vi "PDF Protokoll EPA1065_308 T90.vi"(8 "error in (no error)":errorcluster caption="Fehler (Eingang, kein Fehler)") -> (0 "error out":errorcluster caption="Fehler (Ausgang)")   [LabVIEW 2020, in "EPA 1065.lvlib" / "T90 Test 1065-308.lvlib"]
uses:
  T90 Test 1065-308.lvlib
  Ergebnis.ctl
  Modus.ctl
  Aktion FGV T90.ctl
  Seiten/FT-IR/FGV FT-IR Gasliste Aktionen.ctl
  Seiten/FT-IR/FGV FT-IR Aktionen.ctl
  Seiten/System Einstellungen V2/Aktioen FGV System Konstanten.ctl
  Sprachverwaltung/FGV Aktion Tabelle zerlegen.ctl
  Aktion FGV Datenmanagment.ctl
  Seiten/Anlagengrenzwerte/FGV Anlagengrenzwerte Aktionen.ctl
  <vilib>/Utility/miscctls.llb/LVPrintingMarginsTypeDef.ctl
  Allgemein/allgemeine Sub-VIs.lvlib
  Seiten/FT-IR/FT-IR.lvlib
  Seiten/System Einstellungen V2/System Einstellungen V2.lvlib
  Seiten/Anlagengrenzwerte/Anlagengrenzwerte.lvlib
  Sprachverwaltung/Sprachverwaltung.lvlib
panel:
  out "Modus":string caption="Mode:"
  in  "Modus":T1 caption="Modus:" items=["CG zu PNS", "CG zu Entnahmestelle"]
  out "Einheit 2":string caption="Einheit"
  out "Durchfluss FT-IR:":string caption="Flow FTIR:"
  out "Frequenz 2":string
  out "Frequenz 1":string
  out "Versa Serial number:":string caption="Serial number:"
  out "Anlage:":string caption="Measuring Device:"
  out "Methode (Recipe):":string
  out "Date & Time:":string
  out "Accuracy:":string
  out "Gas Bottle Nr.:":string
  out "Ergebnis 4":T2
  out "Ergebnis 3":T2
  out "Ergebnis 2":T2
  out "Ergebnis 1":T2
  out "Averaged T90-T10 2":string caption="Averaged T90-T10"
  out "Averaged T10-T90 2":string caption="Averaged T10-T90"
  out "Ergebnis x5 (T90 T10)":string caption="Mean T10-T90"
  out "Ergebnis x5 (T10 T90)":string caption="Mean T10-T90"
  out "Averaged T90-T10":string
  out "Averaged T10-T90":string
  out "T90 Result":waveform(sgl)(graph) caption="T90"
  out "Tabelle":string[][](table)
  out "Ergebnis:":string caption="Result:"
  out "Konzentration:":string caption="Setpoint:"
  out "Komponente:":string caption="Component:"
  out "Bearbeiter:":string caption="Editor:"
  out "Serial number:":string
  out "Messgerät:":string caption="Analyzer:"
  # "T90 EPA § 1065.308"
  # "Limits"
  # "Result"
  # "s"
  # ">5"
  # "s"
  # ">5"
  # "s"
  # "<10s"
  # "s"
  # "<10s"
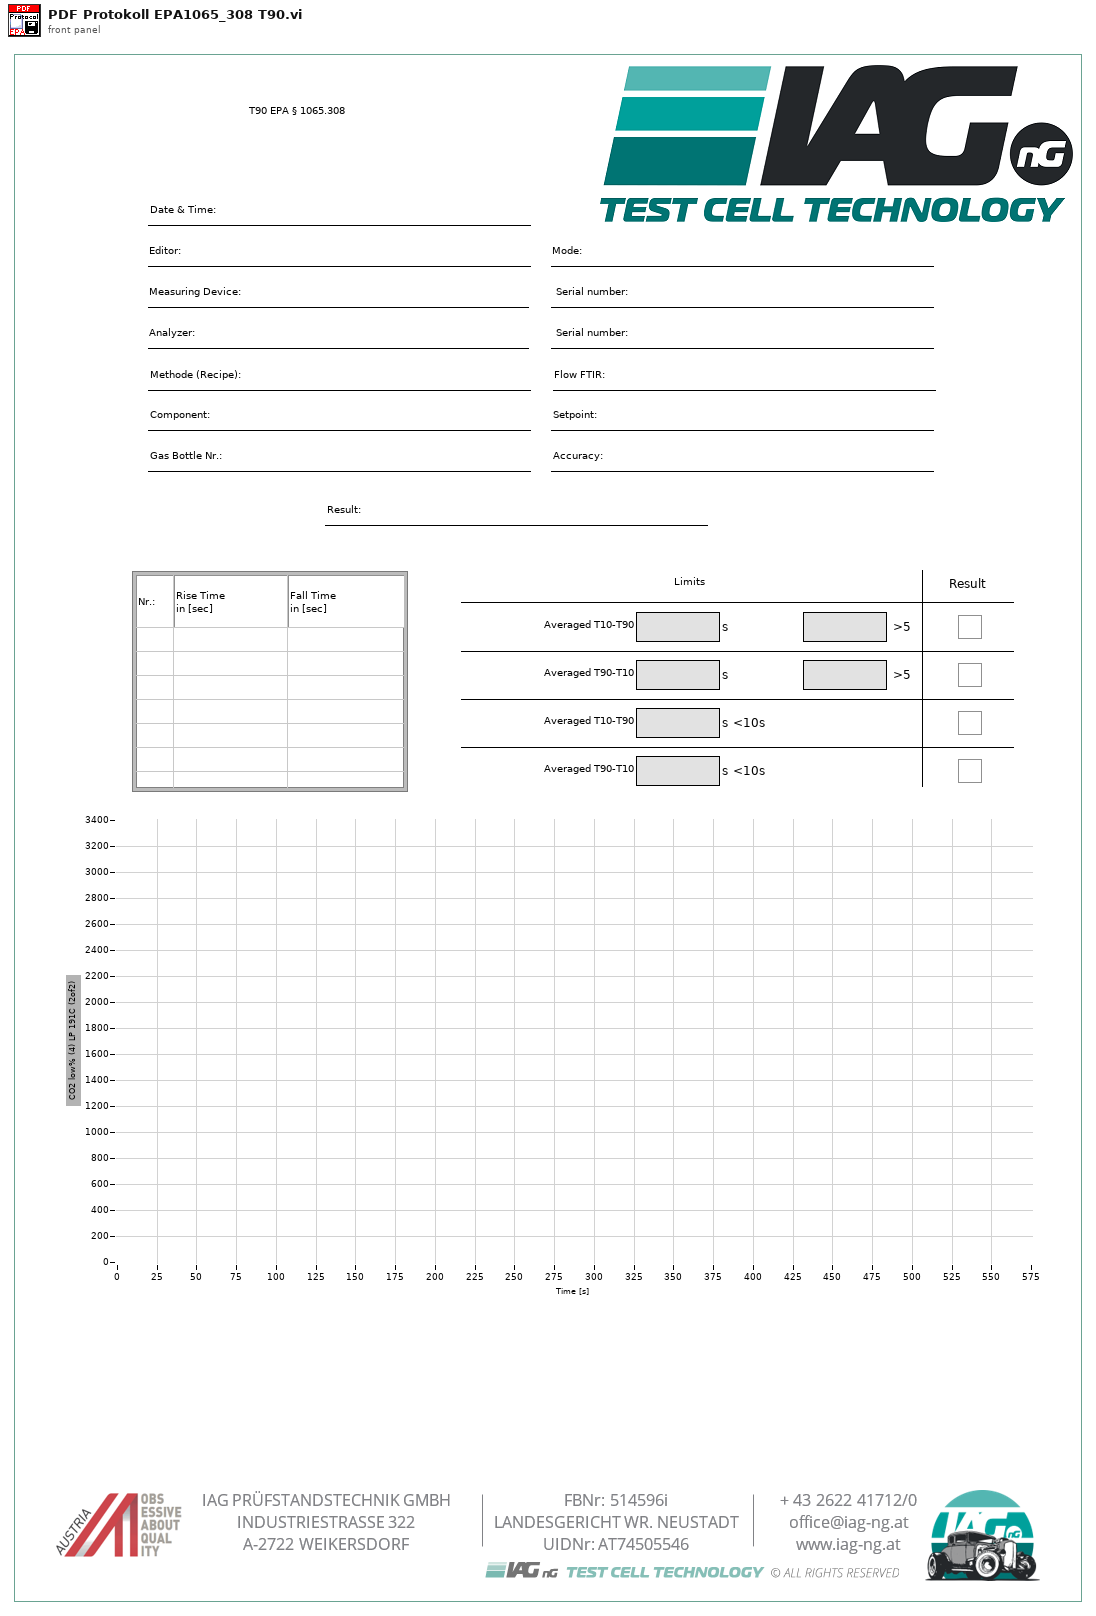
[diagram p1: front panel]
types:
  T1 = typedef "EPA 1065.lvlib/T90 Test 1065-308.lvlib/Modus.ctl" = u16
  T2 = typedef "EPA 1065.lvlib/T90 Test 1065-308.lvlib/Ergebnis.ctl" = bool
  T3 = typedef "Sprachverwaltung.lvlib/FGV Aktion Tabelle zerlegen.ctl" = enum16{"laden", "vereinzeln", "speichern"}
  T4 = typedef "System Einstellungen V2.lvlib/Aktioen FGV System Konstanten.ctl" = enum16{"lesen", "laden", "speichern", "Sprache"}
  T5 = typedef "FT-IR.lvlib/FGV FT-IR Aktionen.ctl" = enum16{"lesen", "NOG setzen", "NOS setzen", "Initialisieren", "speichern", "ALLES setzen", "FT-IR Spektrum loggen", "Komm Stoppen", "Spektrum LogKonfig"}
  T6 = typedef "FT-IR.lvlib/FGV FT-IR Gasliste Aktionen.ctl" = enum16{"lesen", "Gasliste FT-IR", "Gasliste ausgelesen", "laden", "speichern", "löschen"}
  T7 = typedef "EPA 1065.lvlib/T90 Test 1065-308.lvlib/Aktion FGV T90.ctl" = enum16{"lesen", "Konfig Daten", "speichern", "laden", "T90 aktiv", "T90 inaktiv", "Ext. Ventil aktivieren", "Ext. Ventil deaktivieren", "N2 spülen aktiv", "N2 spülen inaktiv", "Ergebnis Textfile"}
  T8 = typedef "EPA 1065.lvlib/T90 Test 1065-308.lvlib/Aktion FGV Datenmanagment.ctl" = enum16{"init", "lesen", "Istwerte schreiben", "höchsten Peak setzen", "Auswerten", "Grenzen setzen", "Sollwert ändern", "Rise T10", "Rise T90", "Fall T90", "Fall T10", "Bit löschen", "Umschaltzeitpunkt"}
  T9 = typedef "Anlagengrenzwerte.lvlib/FGV Anlagengrenzwerte Aktionen.ctl" = enum16{"Lesen", "Grenzwerte schreiben"}
  T10 = enum32{"Portrait", "Landscape", "Rotated Portrait", "Rotated Landscape"}
  T11 = typedef "LVPrintingMarginsTypeDef.ctl" = cluster{"Top":sgl, "Left":sgl, "Bottom":sgl, "Right":sgl, "Measurement System":enum8{"Inches", "cm"}}
  T12 = typedef "EPA 1065.lvlib/T90 Test 1065-308.lvlib/T90 Konfig Daten.ctl" = cluster{"Bearbeiter:":string, "Komponente:":u16, "Gasflaschen Nr.:":string, "Accuracy":dbl, "Sollwert":dbl, "Modus":T1, "Abschaltzeit:":dbl, "Abweichung:":dbl, "Pfad:":path, "Textname:":string, "CG Aufschaltzeit:":dbl, "Einheit":string, "N2 Aufschaltzeit:":dbl, "Analysator":T13, "Gasflasche":T14, "Konfig Gasflasche":T15, "Frequency:":T16}
  T13 = typedef "System Einstellungen V2.lvlib/Analysatoren.ctl" = string
  T14 = typedef "System Einstellungen V2.lvlib/Gasflasche Auswahl.ctl" = u16
  T15 = typedef "System Einstellungen V2.lvlib/Konfig Gasflasche.ctl" = bool
  T16 = typedef "EPA 1065.lvlib/T90 Test 1065-308.lvlib/Frequenz.ctl" = u16
  T17 = cluster{"Modell":string, "ProjektNummer":string, "Software Version":string, "Seriennummer":string}
  T18 = typedef "String - Ausgabefeld.ctl" = string
  T19 = typedef "EPA 1065.lvlib/T90 Test 1065-308.lvlib/Datencluster.ctl" = cluster{"Höchster Peak":T20, "T10 Grenzwert":T20, "T90 Grenzwert":T20, "Rise Times":dbl[], "Fall Times":dbl[], "RiseTime gemittelt":T20, "FallTime gemittelt":T20, "Zeitstempel":timestamp[], "Rise T10":bool, "Rise T90":bool, "Fall T10":bool, "Fall T90":bool, "RiseTime >5":bool, "Falltime >5":bool, "RiseTime <10":bool, "Falltime <10":bool, "T0-T90":dbl[], "T100-T10":dbl[]}
  T20 = typedef "Zahlen-Eingabefeld.ctl" = sgl
  T21 = typedef "Anlagengrenzwerte.lvlib/Anlagen-Grenzwerte Anzeige.ctl" = cluster{"Eingangsdruck FT-IR:":T22, "Durchfluss FT-IR:":T22, "Durchfluss CalGas:":T22, "Druck Ausgang:":T22, "Druck Kalter Block:":T22, "Heizleitungen intern:":T22, "Heizleitung zu FT-IR:":T22, "Heizung Filterblock:":T22, "Heizung Pumpe:":T22, "Heizleitung Extern SP1:":T22, "Heizleitung Extern SP2:":T22, "FT-IR Heizung Messzelle:":T22, "Schaltschranktemperatur:":T22, "Gaskühler:":T22}
  T22 = typedef "Anlagengrenzwerte.lvlib/Anlagen-Parameter Anzeige.ctl" = cluster{"Sollwert":sgl, "Warn-Min":sgl, "Warn-Max":sgl, "Abschalt-Min":sgl, "Abschalt-Max":sgl, "Regler":u16}
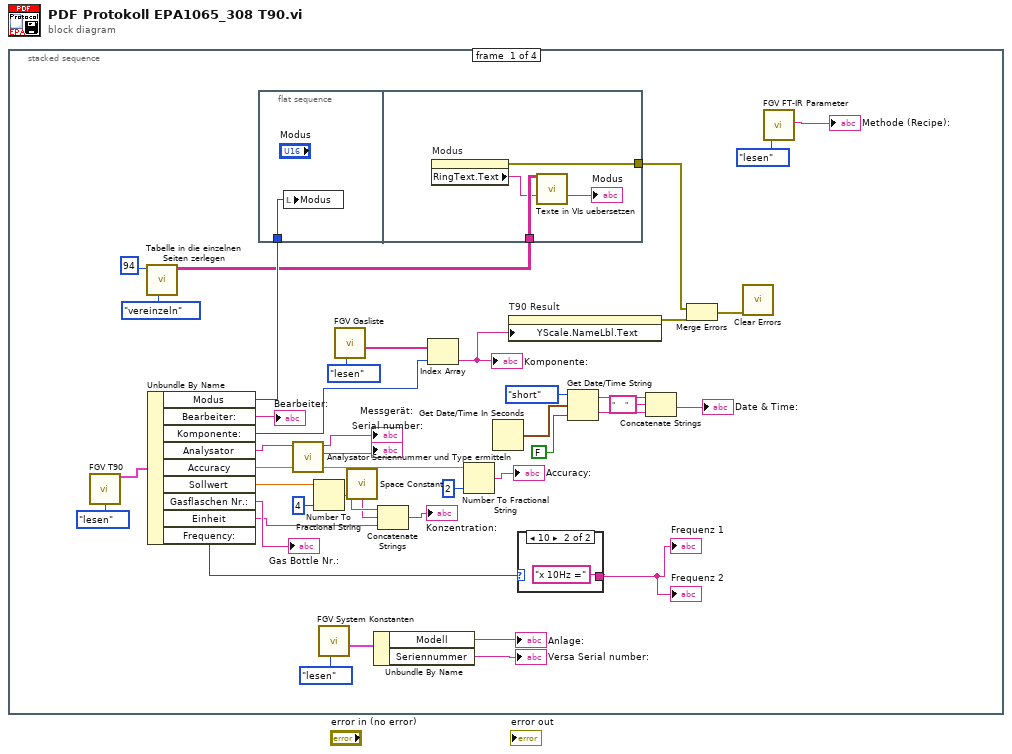
[diagram p0: block diagram]
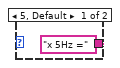
[diagram p2: hidden frame]
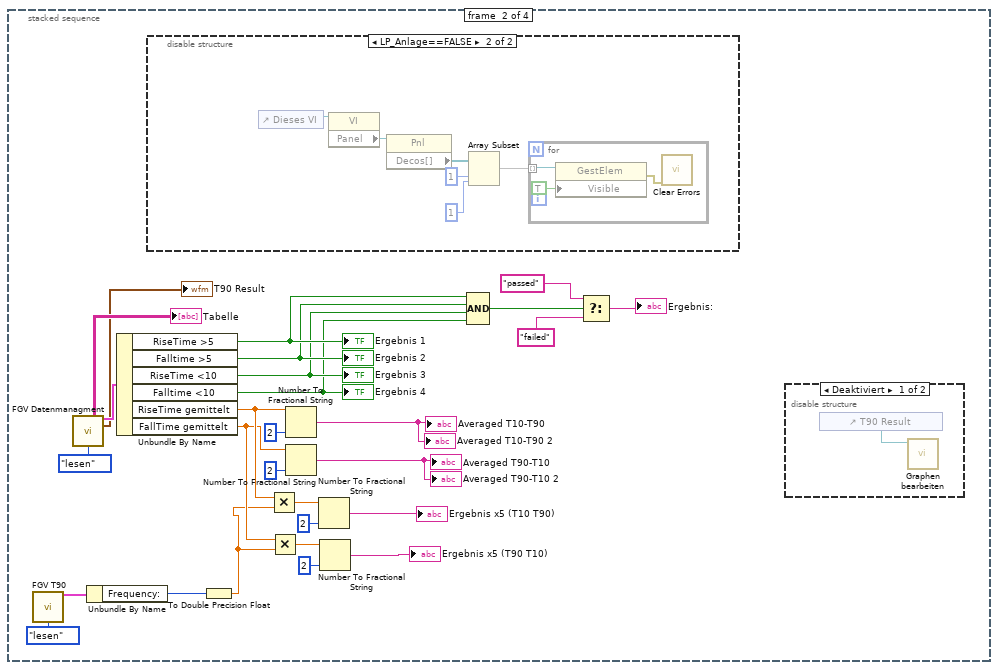
[diagram p3: hidden frame]
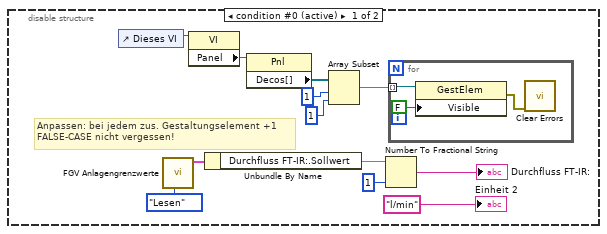
[diagram p4: hidden frame]
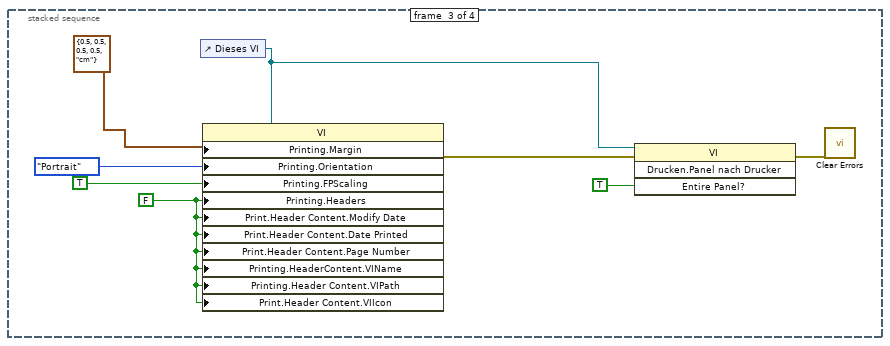
[diagram p6: hidden frame]
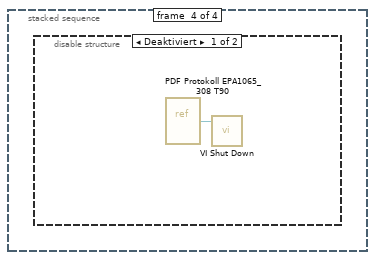
[diagram p7: hidden frame]
diagram:
  n1 = stacked-sequence {
    frame #0 {
      n2 = call "FGV T90.vi"("Aktion"=Aktion_FGV_T90."lesen") -> ("T90 Konfig Daten"=w34:T12)  [unwired: 9 in, 5 out]
      n3 = call "Tabelle in die einzelnen Seiten zerlegen.vi"("Aktion"=FGV_Aktion_Tabelle_zerlegen."vereinzeln", "Index (Seite)"=94) -> ("Sprachliste"=w3:string[][])  [unwired: 7 in, 2 out]
      n4 = Unbundle By Name(w34) -> ("Modus"=w9:T1, "Bearbeiter:"=→"Bearbeiter:":string, "Komponente:"=w30:u16, "Analysator"=w12:T13, "Accuracy"=w27:dbl, "Sollwert"=w23:dbl, "Gasflaschen Nr.:"=→"Gas Bottle Nr.:":string, "Einheit"=w17:string, "Frequency:"=w11:T16)
      n5 = flat-sequence {
        tunnel: w9 -> [w43]
        tunnel: [w47] -> w7
        tunnel: w3 -> [w46]
        frame #0 {
          n6 = local write "Modus"(w43) -> ()
        }
        frame #1 {
          n7 = property on="Modus" class="Ring (strikt)"() -> (error out=w47:errorcluster, "RingText.Text"=w45:string)  [unwired: 2 in, 1 out]
          n8 = call "Texte in VIs uebersetzen.vi"("Sprachliste"=w46, "String zum Übersetzen"=w45) -> ("String zum Übersetzen"=→"Modus":string)  [unwired: 9 in, 4 out]
        }
      }
      n9 = call "Analysator Seriennummer und Type ermitteln.vi"("Analysator"=w12) -> ("Type"=→"Serial number:":string, "Name für Protokoll"=→"Messgerät:":string)  [unwired: 8 in, 1 out]
      n10 = Number To Fractional String(number=w23, precision (6)=i16 4 ("Genauigkeit (6)")) -> (F-format string=w20:string)  [unwired: 2 in]
      n11 = call "FGV System Konstanten.vi"("Aktionen"=Aktioen_FGV_System_Konstanten."lesen") -> ("Cluster out"=w15:T17)  [unwired: 6 in, 4 out]
      n12 = call "FGV Gasliste.vi"("Aktionen"=FGV_FT-IR_Gasliste_Aktionen."lesen") -> ("Aktuelle Gasliste gesamt"=w31:T18[])  [unwired: 8 in, 2 out]
      n13 = call <vilib>:"Space Constant.vi"() -> ("String"=w18:string)
      n14 = Unbundle By Name(w15) -> ("Modell"=→"Anlage:":string, "Seriennummer"=→"Versa Serial number:":string)
      n15 = Concatenate Strings(w20, w18, w17) -> (→"Konzentration:":string)
      n16 = Index Array(array=w31, index=w30) -> (element=w21:T18)
      "Komponente:" <- w21
      n17 = Number To Fractional String(number=w27, precision (6)=i16 2 ("Genauigkeit (6)")) -> (F-format string=→"Accuracy:":string)  [unwired: 2 in]
      n18 = Get Date/Time In Seconds() -> (seconds since 1Jan1904=w42:timestamp)
      n19 = property on="T90 Result" class="SVGraph (strikt)"("YScale.NameLbl.Text"=w21) -> (error out=w8:errorcluster)  [unwired: 2 in, 1 out]
      n20 = case shown="10" w11 {
        tunnel: ["x 5Hz =" "x 10Hz ="] -> w10
        frame 5, Default {
        }
        frame 10 {
        }
      }
      "Frequenz 1" <- w10
      "Frequenz 2" <- w10
      n21 = Get Date/Time String(date format (0)=enum16{"short", "long", "abbreviated"}."short" ("Datumsformat (0)"), seconds (now)=w42, want seconds? (F)=FALSE ("Angabe von Sekunden? (F)")) -> (date string=w41:string, time string=w40:string)
      n22 = Concatenate Strings(w41, "     " ("String"), w40) -> (→"Date & Time:":string)
      n23 = Merge Errors(w7, w8) -> (w6:errorcluster)
      n24 = call <vilib>:"Clear Errors.vi"("error in (no error)"=w6) -> ()  [unwired: 5 in, 2 out]
      n25 = call "FGV FT-IR Parameter.vi"("Aktion"=FGV_FT-IR_Aktionen."lesen") -> ("Current Recipe"=→"Methode (Recipe):":string)  [unwired: 11 in, 7 out]
    }
    frame #1 {
      n26 = call "FGV T90.vi"("Aktion"=Aktion_FGV_T90."lesen") -> ("T90 Konfig Daten"=w52:T12)  [unwired: 9 in, 5 out]
      n27 = call "FGV Datenmanagment.vi"("Aktion"=Aktion_FGV_Datenmanagment."lesen") -> ("Ergebnistabelle"=→"Tabelle":string[][], "Daten"=w75:T19, "T90 Signalverlauf"=→"T90 Result":waveform(sgl))  [unwired: 7 in, 5 out]
      n28 = Unbundle By Name(w52) -> ("Frequency:"=w51:T16)
      n29 = Unbundle By Name(w75) -> ("RiseTime >5"=w58:bool, "Falltime >5"=w57:bool, "RiseTime <10"=w56:bool, "Falltime <10"=w55:bool, "RiseTime gemittelt"=w68:T20, "FallTime gemittelt"=w67:T20)
      "Ergebnis 4" <- w55
      "Ergebnis 3" <- w56
      "Ergebnis 2" <- w57
      "Ergebnis 1" <- w58
      n30 = disable-structure shown="LP_Anlage==FALSE" {
        frame condition #0 (active) {
          # "Anpassen: bei jedem zus. Gestaltungselement +1\nFALSE-CASE nicht vergessen!"
          n31 = control-ref of="Dieses VI"() -> (w85:refnum<vi>)
          n32 = call "FGV Anlagengrenzwerte.vi"("Aktion"=FGV_Anlagengrenzwerte_Aktionen."Lesen") -> ("Anlagen-Grenzwerte Anzeige"=w87:T21)  [unwired: 1 in, 9 out]
          n33 = property class="VI"(reference=w85) -> ("Panel"=w82:refnum<vi>)  [unwired: 1 in, 2 out]
          n34 = Unbundle By Name(w87) -> ("Durchfluss FT-IR:.Sollwert"=w86:sgl)
          n35 = property class="Pnl"(reference=w82) -> ("Decos[]"=w83:refnum<vi>[])  [unwired: 1 in, 2 out]
          n36 = Array Subset(array=w83, index=1 ("Länge"), length=1 ("Länge")) -> (w84:refnum<vi>[])
          n37 = Number To Fractional String(number=w86, precision (6)=i16 1 ("Genauigkeit (6)")) -> (F-format string=→"Durchfluss FT-IR:":string)  [unwired: 2 in]
          n38 = for {
            tunnel: w84 -> [w92] mode=indexing
            n39 = property class="GestElem"(reference=w92, "Visible"=FALSE ("Sichtbar")) -> (error out=w90:errorcluster)  [unwired: 1 in, 1 out]
            n40 = call <vilib>:"Clear Errors.vi"("error in (no error)"=w90) -> ()  [unwired: 5 in, 2 out]
          }
          "Einheit 2" <- "l/min" ("Einheit 2")
        }
        frame condition #1 {
          n41 = control-ref of="Dieses VI"() -> (w98:refnum<vi>)
          n42 = property class="VI"(reference=w98) -> ("Panel"=w95:refnum<vi>)  [unwired: 1 in, 2 out]
          n43 = property class="Pnl"(reference=w95) -> ("Decos[]"=w96:refnum<vi>[])  [unwired: 1 in, 2 out]
          n44 = Array Subset(array=w96, index=1 ("Index"), length=1 ("Länge")) -> (w97:refnum<vi>[])
          n45 = for {
            tunnel: w97 -> [w101] mode=indexing
            n46 = property class="GestElem"(reference=w101, "Visible"=TRUE ("Sichtbar")) -> (error out=w99:errorcluster)  [unwired: 1 in, 1 out]
            n47 = call <vilib>:"Clear Errors.vi"("error in (no error)"=w99) -> ()  [unwired: 5 in, 2 out]
          }
        }
      }
      n48 = To Double Precision Float(number=w51) -> (double precision float=w50:dbl)
      n49 = Multiply(x=w68, y=w50) -> (x*y=w72:dbl)
      n50 = Multiply(x=w67, y=w50) -> (x*y=w71:dbl)
      n51 = Number To Fractional String(number=w68, precision (6)=i16 2 ("Genauigkeit (6)")) -> (F-format string=→"Averaged T10-T90 2" →"Averaged T10-T90":string)  [unwired: 2 in]
      n52 = Number To Fractional String(number=w67, precision (6)=i16 2 ("Genauigkeit (6)")) -> (F-format string=→"Averaged T90-T10 2" →"Averaged T90-T10":string)  [unwired: 2 in]
      n53 = Number To Fractional String(number=w72, precision (6)=i16 2 ("Genauigkeit (6)")) -> (F-format string=→"Ergebnis x5 (T10 T90)":string)  [unwired: 2 in]
      n54 = Number To Fractional String(number=w71, precision (6)=i16 2 ("Genauigkeit (6)")) -> (F-format string=→"Ergebnis x5 (T90 T10)":string)  [unwired: 2 in]
      n55 = Compound Arithmetic op=AND ("Mehrfacharithmetik")(w58, w57, w56, w55) -> (w54:bool)
      n56 = Select(t="passed", s=w54, f="failed") -> (s? t:f=→"Ergebnis:":string)
      n57 = disable-structure shown="Deaktiviert" {
        frame Disabled {
          n58 = control-ref of="T90 Result"() -> (w102:refnum<vi>)
          n59 = call "Graphen bearbeiten.vi"("T90 Result"=w102) -> ()  [unwired: 10 in, 1 out]
        }
        frame Enabled {
        }
      }
    }
    frame #2 {
      w106 = FALSE ("Drucken:Kopfzeilen?")
      n60 = control-ref of="Dieses VI"() -> (w103:refnum<vi>)
      n61 = property class="VI"(reference=w103, "Printing.Margin"=T11 {"Top"=0.5, "Left"=0.5, "Bottom"=0.5, "Right"=0.5, "Measurement System"=enum."cm"} ("Drucken:Ränder"), "Printing.Orientation"=T10."Portrait" ("Drucken:Seitenausrichtung"), "Printing.FPScaling"=TRUE ("Drucken:Frontpanel-Skalierung?"), "Printing.Headers"=w106, "Print.Header Content.Modify Date"=w106, "Print.Header Content.Date Printed"=w106, "Print.Header Content.Page Number"=w106, "Printing.HeaderContent.VIName"=w106, "Printing.Header Content.VIPath"=w106, "Print.Header Content.VIIcon"=w106) -> (error out=w110:errorcluster)  [unwired: 1 in, 1 out]
      n62 = invoke class="VI" method="Drucken.Panel nach Drucker"(reference=w103, error in=w110, "Entire Panel?"=TRUE ("Abschnittskopfzeilen?")) -> (error out=w104:errorcluster)  [unwired: 1 in, 3 out]
      n63 = call <vilib>:"Clear Errors.vi"("error in (no error)"=w104) -> ()  [unwired: 5 in, 2 out]
    }
    frame #3 {
      n64 = disable-structure shown="Deaktiviert" {
        frame Disabled {
          n65 = vi-ref "PDF Protokoll EPA1065_308 T90.vi"() -> (w111:refnum<vi>)
          n66 = call "VI Shut Down.vi"("VI Referenz"=w111) -> ()  [unwired: 11 in]
        }
        frame Enabled {
        }
      }
    }
  }
